vi "Teleop.vi"(10 "Match Info":T1={"Autonomous Elapsed Seconds"=0.0, "TeleOp Elapsed Seconds"=0.0, "Disabled Elapsed Seconds"=0.0, "Visited Autonomous"=FALSE, "Visited TeleOp"=FALSE, "Visited Disabled"=FALSE, "Autonomous Settings"={"Autonomous Style"=enum."Independent", "VI Refnum"=refnum}}, 11 "Call Context":T2) -> ()   [LabVIEW 2015]
doc: "This VI is called for each TeleOp packet received from the DS where the robot is not disabled. It is often used to read from the joysticks and update I/O or to update setpoints for timed control loops. It should complete and return within 20 milliseconds or it may miss DS packets."
uses:
  Robot Global Data.vi
  <vilib>/Rock Robotics/WPI/DriverStation/WPI_DriverStationMatch Info.ctl
  <vilib>/Rock Robotics/WPI/DriverStation/WPI_DriverStationDerivedRobotMode.ctl
panel:
  out "Boolean 2":bool
  out "Boolean 1":bool
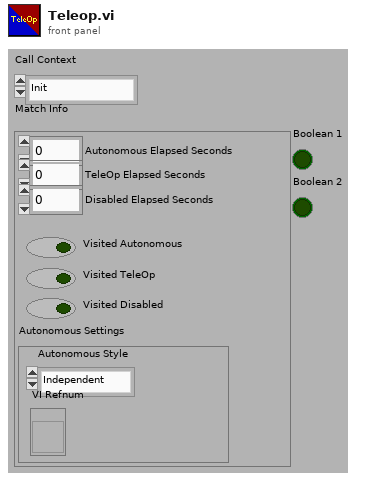
[diagram p1: front panel]
types:
  T1 = typedef "WPI_DriverStationMatch Info.ctl" = cluster{"Autonomous Elapsed Seconds":dbl, "TeleOp Elapsed Seconds":dbl, "Disabled Elapsed Seconds":dbl, "Visited Autonomous":bool, "Visited TeleOp":bool, "Visited Disabled":bool, "Autonomous Settings":cluster{"Autonomous Style":enum16{"Iterative", "Independent"}, "VI Refnum":refnum<vi>}}
  T2 = typedef "WPI_DriverStationDerivedRobotMode.ctl" = enum16{"Init", "Execute", "Stop"}
  T3 = typedef "WPI_JoystickDevRef.ctl" = cluster{"Device":T4}
  T4 = typedef "WPI_JoystickDeviceEnum.ctl" = enum16{"USB 0", "USB 1", "USB 2", "USB 3", "USB 4", "USB 5"}
  T5 = cluster{"axis 1 (x)":dbl, "axis 2 (y)":dbl, "axis 3 (throttle)":dbl, "axis 4":dbl, "axis 5":dbl, "axis 6":dbl}
  T6 = cluster{"Button 1":bool, "Button 2":bool, "Button 3":bool, "Button 4":bool, "Button 5":bool, "Button 6":bool, "Button 7":bool, "Button 8":bool, "Button 9":bool, "Button 10":bool, "Button 11":bool, "Button 12":bool}
  T7 = cluster{"Reverse":bool, "Speed":dbl, "Left":dbl, "Right":dbl}
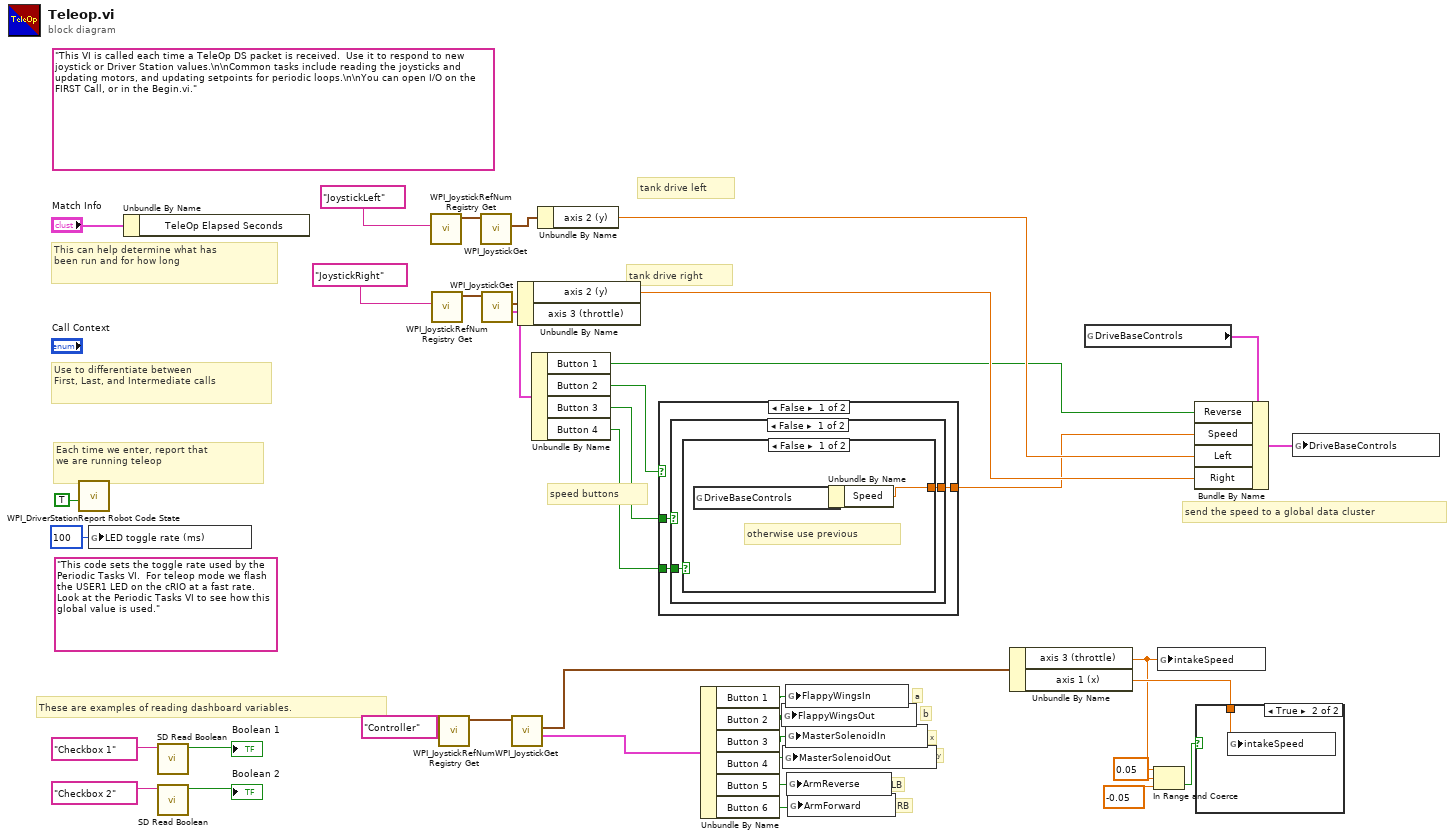
[diagram p0: block diagram]
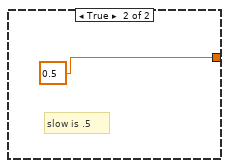
[diagram p2: hidden frame]
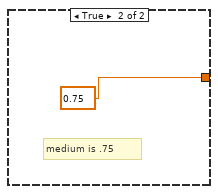
[diagram p3: hidden frame]
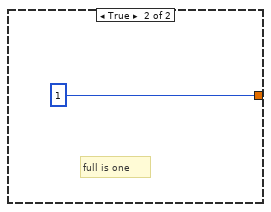
[diagram p4: hidden frame]
diagram:
  (unwired) "This code sets the toggle rate used by the Periodic Tasks VI.  For teleop mode we flash the USER1 LED on the cRIO at a fast rate.  Look at the Periodic Tasks VI to see how this global value is used."
  (unwired) "This VI is called each time a TeleOp DS packet is received.  Use it to respond to new joystick or Driver Station values.\n\nCommon tasks include reading the joysticks and updating motors, and updating setpoints for periodic loops.\n\nYou can open I/O on the FIRST Call, or in the Begin.vi."
  # "send the speed to a global data cluster"
  # "speed buttons"
  # "y"
  # "x"
  # "b"
  # "a"
  # "RB"
  # "LB"
  # "tank drive right"
  # "tank drive left"
  # "These are examples of reading dashboard variables."
  # "Each time we enter, report that\nwe are running teleop"
  # "Use to differentiate between\nFirst, Last, and Intermediate calls"
  # "This can help determine what has\nbeen run and for how long"
  n1 = call <vilib>:"WPI_DriverStationReport Robot Code State.vi"("TeleOp"=TRUE ("Autonomous")) -> ()  [unwired: 10 in, 1 out]
  n2 = global write "Robot Global Data.vi" "LED toggle rate (ms)"(u32 100 ("LED ms toggle rate")) -> ()
  n3 = Unbundle By Name("Match Info") -> ()  [unwired: 1 out]
  n4 = call <vilib>:"SD Read Boolean.vi"("Name"="Checkbox 1" ("refnum name")) -> ("Boolean"=→"Boolean 1":bool)  [unwired: 8 in, 2 out]
  n5 = call <vilib>:"SD Read Boolean.vi"("Name"="Checkbox 2" ("refnum name")) -> ("Boolean"=→"Boolean 2":bool)  [unwired: 8 in, 2 out]
  n6 = call <vilib>:"WPI_JoystickRefNum Registry Get.vi"("refnum name"="JoystickLeft") -> ("JoystickDevRef"=w30:T3)  [unwired: 1 in, 9 out]
  n7 = call <vilib>:"WPI_JoystickRefNum Registry Get.vi"("refnum name"="JoystickRight") -> ("JoystickDevRef"=w27:T3)  [unwired: 1 in, 9 out]
  n8 = call <vilib>:"WPI_JoystickRefNum Registry Get.vi"("refnum name"="Controller") -> ("JoystickDevRef"=w22:T3)  [unwired: 1 in, 9 out]
  n9 = call <vilib>:"WPI_JoystickGet.vi"("JoystickDevRef"=w30) -> ("Axes"=w29:T5)  [unwired: 1 in, 5 out]
  n10 = call <vilib>:"WPI_JoystickGet.vi"("JoystickDevRef"=w27) -> ("Buttons"=w25:T6, "Axes"=w26:T5)  [unwired: 1 in, 4 out]
  n11 = call <vilib>:"WPI_JoystickGet.vi"("JoystickDevRef"=w22) -> ("Buttons"=w21:T6, "Axes"=w17:T5)  [unwired: 1 in, 4 out]
  n12 = Unbundle By Name(w26) -> ("axis 2 (y)"=w23:dbl)  [unwired: 1 out]
  n13 = Unbundle By Name(w25) -> ("Button 1"=w1:bool, "Button 2"=w7:bool, "Button 3"=w6:bool, "Button 4"=w5:bool)
  n14 = Unbundle By Name(w29) -> ("axis 2 (y)"=w24:dbl)
  n15 = case shown="False" w7 {
    tunnel: w6 -> [w41 _]
    tunnel: w5 -> [w40 _]
    tunnel: [w39 1] -> w2
    frame False {
      n16 = case shown="False" w41 {
        tunnel: w40 -> [w43 _]
        tunnel: [w42 0.75] -> w39
        frame False {
          n17 = case shown="False" w43 {
            tunnel: [w44 0.5] -> w42
            frame False {
              # "otherwise use previous"
              n18 = global read "Robot Global Data.vi" "DriveBaseControls"() -> (w45:T7)
              n19 = Unbundle By Name(w45) -> ("Speed"=w44:dbl)
            }
            frame True {
              # "slow is .5"
            }
          }
        }
        frame True {
          # "medium is .75"
        }
      }
    }
    frame True {
      # "full is one"
    }
  }
  n20 = Unbundle By Name(w21) -> ("Button 1"=w11:bool, "Button 2"=w10:bool, "Button 3"=w9:bool, "Button 4"=w8:bool, "Button 5"=w18:bool, "Button 6"=w19:bool)
  n21 = global write "Robot Global Data.vi" "FlappyWingsOut"(w10) -> ()
  n22 = global write "Robot Global Data.vi" "MasterSolenoidOut"(w8) -> ()
  n23 = global write "Robot Global Data.vi" "FlappyWingsIn"(w11) -> ()
  n24 = global write "Robot Global Data.vi" "MasterSolenoidIn"(w9) -> ()
  n25 = global write "Robot Global Data.vi" "ArmReverse"(w18) -> ()
  n26 = global write "Robot Global Data.vi" "ArmForward"(w19) -> ()
  n27 = Unbundle By Name(w17) -> ("axis 3 (throttle)"=w13:dbl, "axis 1 (x)"=w16:dbl)
  n28 = global read "Robot Global Data.vi" "DriveBaseControls"() -> (w3:T7)
  n29 = In Range and Coerce(upper limit=0.05, x=w13, lower limit=-0.05) -> (In Range?=w12:bool)  [unwired: 1 out]
  n30 = global write "Robot Global Data.vi" "intakeSpeed"(w13) -> ()
  n31 = Bundle By Name(cluster=w3, "Reverse"=w1, "Speed"=w2, "Left"=w24, "Right"=w23) -> (w4:T7)
  n32 = case shown="True" w12 {
    tunnel: w16 -> [_ w49]
    frame False {
    }
    frame True {
      n33 = global write "Robot Global Data.vi" "intakeSpeed"(w49) -> ()
    }
  }
  n34 = global write "Robot Global Data.vi" "DriveBaseControls"(w4) -> ()
